vi "Main On Load Action VI.vi"(8 "error in (no error)":errorcluster, 11 "Device Item Ref in":T1 format="%.0x") -> (0 "error out":errorcluster, 3 "Device Item Ref out":T1 format="%.0x")   [LabVIEW 2011, in "Engine Sim System Explorer.lvlib"]
uses:
  Engine Sim System Explorer.lvlib
  <vilib>/NI Veristand/Custom Device API/Custom Device API.lvlib
  <vilib>/NI Veristand/Custom Device API/Custom Device Loop Type.ctl
  <vilib>/NI Veristand/Custom Device API/Custom Device Channel Type.ctl
  <vilib>/NI Veristand/Custom Device API/Custom Device Channel.ctl
  Shared/Engine Simulation Global.vi
  Engine Simulation Shared.lvlib
  <vilib>/NI Veristand/Custom Device API/Get Item Property (Dependent File).vi
  <vilib>/NI Veristand/Custom Device API/Set Item Property (Path).vi
  <vilib>/NI Veristand/Custom Device Tools/Custom Device Utility Library/Custom Device Utility Library.lvlib
  <vilib>/NI Veristand/Custom Device Tools/Custom Device Utility Library/NI VeriStand - Search for Item by GUID.vi
  <vilib>/NI Veristand/Custom Device API/Get Item Property (Boolean).vi
  <vilib>/NI Veristand/Custom Device API/Get Item Property (Dependent Node Pointer).vi
  <vilib>/NI Veristand/Custom Device API/Custom Device Execution Mode.ctl
  <vilib>/NI Veristand/Custom Device API/Path Type.ctl
  <vilib>/NI Veristand/Custom Device API/Path Specification.ctl
  <vilib>/NI Veristand/Custom Device API/Custom Device Supported Target.ctl
  <vilib>/NI Veristand/Custom Device API/Custom Device Path Data.ctl
  NationalInstruments.VeriStand.SystemDefinitionAPI
  <vilib>/NI Veristand/Custom Device API/Custom Device Item Ref.ctl
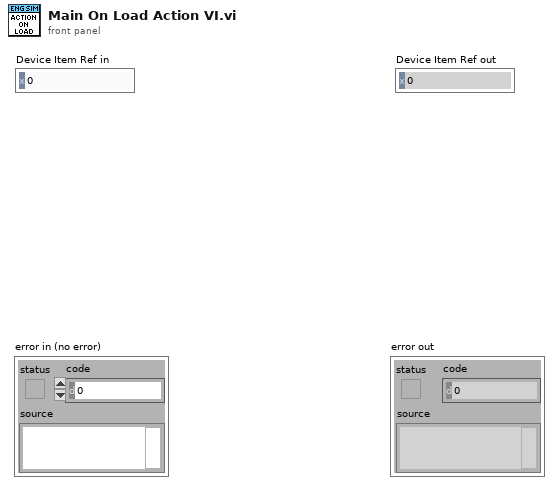
[diagram p1: front panel]
types:
  T1 = typedef "Custom Device API.lvlib/Custom Device Item Ref.ctl" = u64
  T2 = typedef "Custom Device API.lvlib/Custom Device Loop Type.ctl" = enum32{"While Loop", "Timed Loop"}
  T3 = typedef "Custom Device API.lvlib/Custom Device Channel.ctl" = cluster{"Type":T4, "Units":string, "Default Value":dbl, "Faultable":bool, "Scalable":bool}
  T4 = typedef "Custom Device API.lvlib/Custom Device Channel Type.ctl" = enum16{"Input", "Output"}
  T5 = typedef "Custom Device API.lvlib/Path Type.ctl" = enum16{"Absolute", "To Base", "To Common Data Dir", "To Application Data Dir"}
  T6 = typedef "Custom Device API.lvlib/Custom Device Supported Target.ctl" = enum16{"All", "PharLap", "VxWorks", "Windows", "PharLap & Windows", "PharLap & VxWorks", "VxWorks & Windows"}
  T7 = typedef "Custom Device API.lvlib/Custom Device Execution Mode.ctl" = enum16{"Asynchronous", "Inline HW Interface", "Inline Model Interface", "Inline Timing and Sync", "Asynchronous Timing and Sync"}
  T8 = typedef "Custom Device API.lvlib/Dependent File Optional Info.ctl" = cluster{"Version":string, "RTDestination":path, "ForceDownload":bool, "SupportedTarget":string, "MD5":string}
  T9 = typedef "Custom Device API.lvlib/Custom Device Path Data.ctl" = cluster{"SupportedTarget":T6, "Source":T10, "RT Destination":path}
  T10 = typedef "Custom Device API.lvlib/Path Specification.ctl" = cluster{"Path":path, "Type":T5}
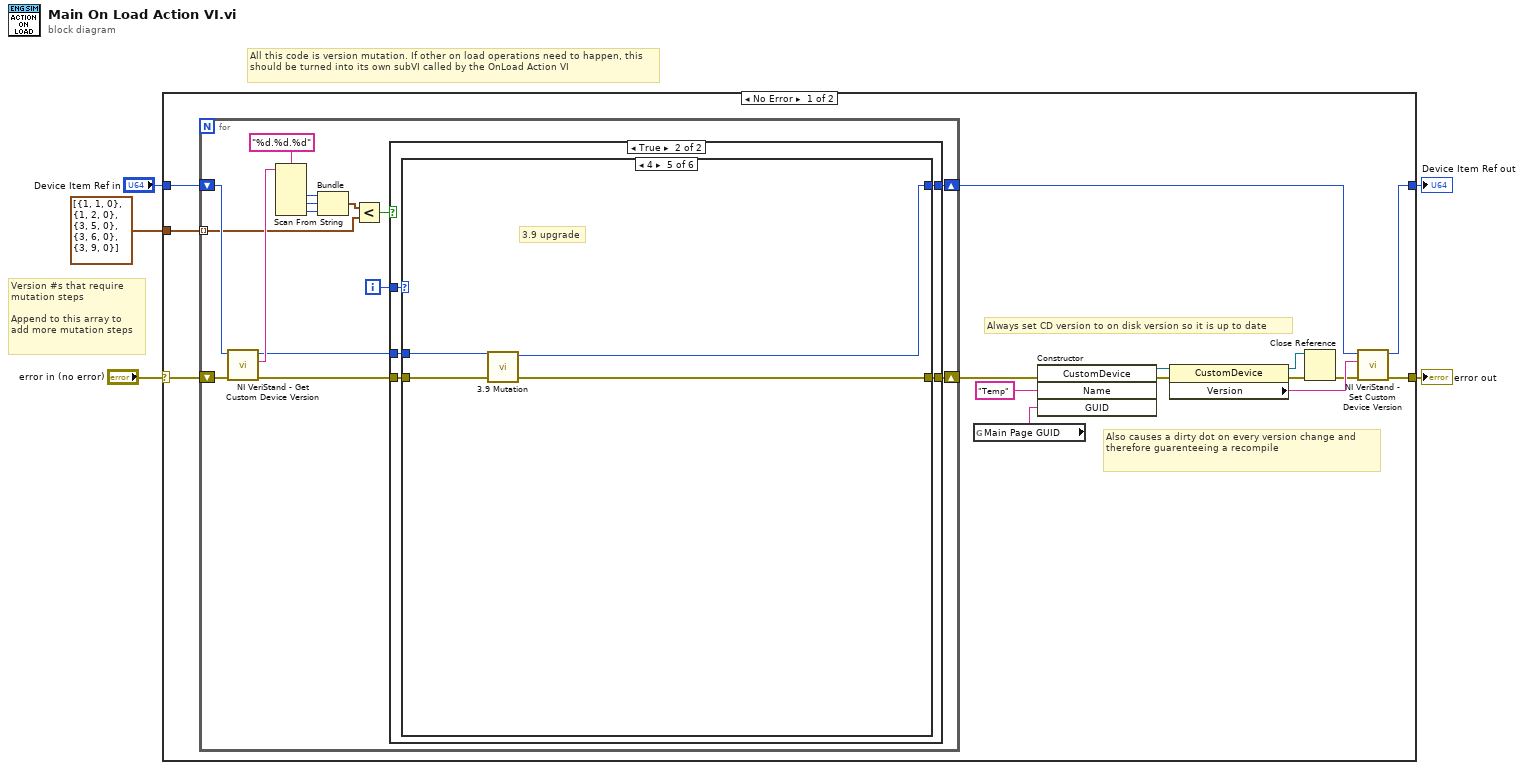
[diagram p0: block diagram]
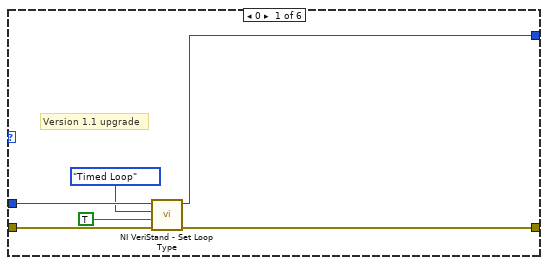
[diagram p3: hidden frame]
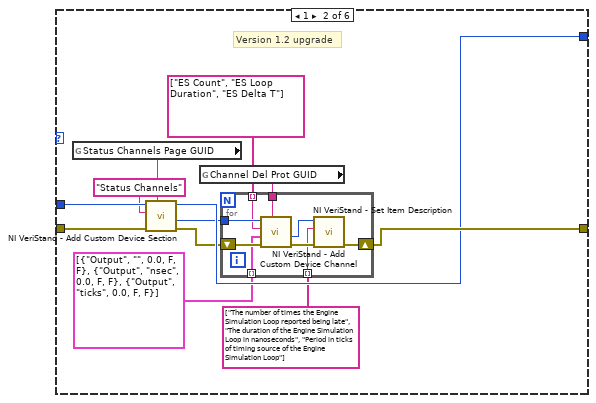
[diagram p4: hidden frame]
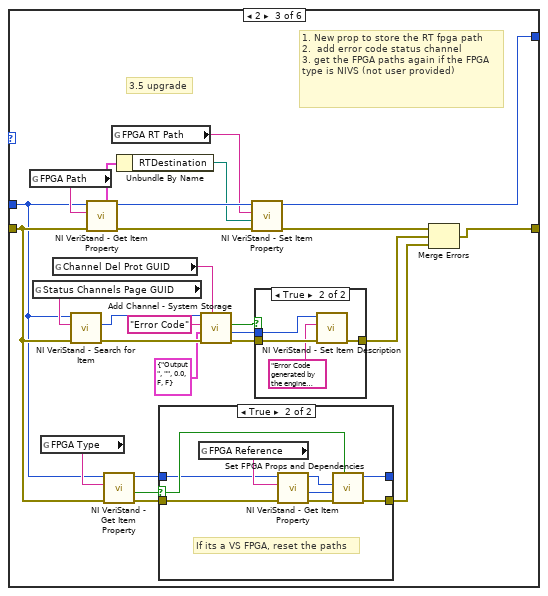
[diagram p5: hidden frame]
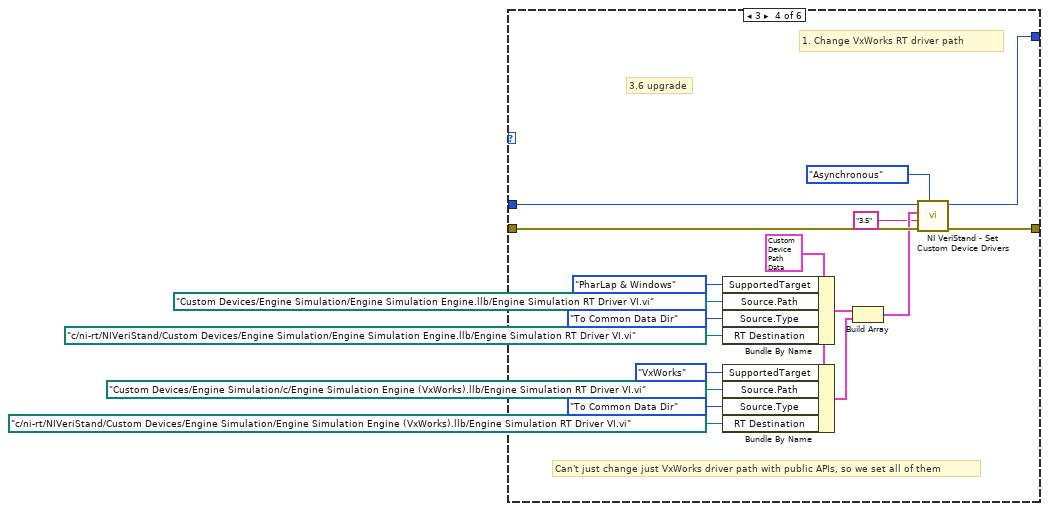
[diagram p8: hidden frame]
diagram:
  # "All this code is version mutation. If other on load operations need to happen, this should be turned into its own subVI called by the OnLoad Action VI"
  # "Version #s that require\nmutation steps\n\nAppend to this array to\nadd more mutation steps"
  n1 = case shown="No Error" "error in (no error)" {
    selector: "error in (no error)" -> [w19 w137]
    tunnel: [w9 w137] -> w4
    tunnel: "Device Item Ref in" -> [w18 w136]
    tunnel: [w7 w136] -> w2
    tunnel: cluster{i32, i32, i32}[] [{1, 1, 0}, {1, 2, 0}, {3, 5, 0}, {3, 6, 0}, {3, 9, 0}] -> [w20 _]
    frame No Error {
      # "Also causes a dirty dot on every version change and therefore guarenteeing a recompile"
      # "Always set CD version to on disk version so it is up to date"
      n2 = for {
        tunnel: w20 -> [w22] mode=indexing
        shift-right: [w26] -> w10
        shift-left: w19 -> [w31]
        shift-right: [w24] -> w8
        shift-left: w18 -> [w30]
        i -> [w23]
        n3 = call <vilib>:"NI VeriStand - Get Custom Device Version.vi"("error in (no error)"=w31, "Device Ref in"=w30) -> ("error out"=w27:errorcluster, "Value"=w29:string, "Device Ref out"=w25:T1)  [unwired: 7 in]
        n4 = Scan From String(format string="%d.%d.%d", input string=w29) -> (output 1=w33:i32, output 2=w34:i32, output 3=w21:i32)  [unwired: 5 in, 3 out]
        n5 = Bundle(w33, w34, w21) -> (w35:cluster{i32, i32, i32})  [unwired: 1 in]
        n6 = Less?(x=w35, y=w22) -> (x < y?=w28:bool)
        n7 = case shown="True" w28 {
          tunnel: w27 -> [w37 w42]
          tunnel: [w37 w41] -> w26
          tunnel: w25 -> [w36 w38]
          tunnel: [w36 w39] -> w24
          tunnel: w23 -> [_ w40]
          frame False {
          }
          frame True {
            n8 = case shown="4" w40 {
              tunnel: w42 -> [w48 w59 w76 w126 w133 w135]
              tunnel: [w45 w60 w70 w129 w131 w135] -> w41
              tunnel: [w46 w56 w89 w128 w130 w134] -> w39
              tunnel: w38 -> [w47 w58 w72 w127 w132 w134]
              frame 0 {
                # "Version 1.1 upgrade"
                n9 = call <vilib>:"NI VeriStand - Set Loop Type.vi"("error in (no error)"=w48, "Use Device Clock (Timed Loops only)"=TRUE, "Loop type"=Custom_Device_Loop_Type."Timed Loop", "Device Ref in"=w47) -> ("error out"=w45:errorcluster, "Device Ref out"=w46:T1)  [unwired: 6 in]
              }
              frame 1 {
                # "Version 1.2 upgrade"
                n10 = global read "Engine Simulation Global.vi" "Status Channels Page GUID"() -> (w49:string)
                n11 = call <vilib>:"NI VeriStand - Add Custom Device Section.vi"("GUID (Default Section)"=w49, "error in (no error)"=w59, "Section Name"="Status Channels", "Parent Ref in"=w58) -> ("error out"=w54:errorcluster, "Section Ptr"=w55:T1, "Parent Ref out"=w56:T1)  [unwired: 4 in, 1 out]
                n12 = global read "Engine Simulation Global.vi" "Channel Del Prot GUID"() -> (w52:string)
                n13 = for {
                  tunnel: w55 -> [w69]
                  shift-right: [w63] -> w60
                  shift-left: w54 -> [w68]
                  tunnel: T3[] [{"Type"=enum."Output", "Units"="", "Default Value"=0.0, "Faultable"=FALSE, "Scalable"=FALSE}, {"Type"=enum."Output", "Units"="nsec", "Default Value"=0.0, "Faultable"=FALSE, "Scalable"=FALSE}, {"Type"=enum."Output", "Units"="ticks", "Default Value"=0.0, "Faultable"=FALSE, "Scalable"=FALSE}] -> [w67] mode=indexing
                  tunnel: w52 -> [w66]
                  tunnel: string[] ["ES Count", "ES Loop Duration", "ES Delta T"] -> [w65] mode=indexing
                  tunnel: string[] ["The number of times the Engine Simulation Loop reported being late", "The duration of the Engine Simulation Loop in nanoseconds", "Period in ticks of timing source of the Engine Simulation Loop"] -> [w62] mode=indexing
                  n14 = call <vilib>:"NI VeriStand - Add Custom Device Channel.vi"("GUID (Default Channel)"=w66, "error in (no error)"=w68, "Channel"=w67, "Channel Name"=w65, "Parent Ref in"=w69) -> ("error out"=w64:errorcluster, "Channel Ref"=w61:T1)  [unwired: 3 in, 2 out]
                  n15 = call <vilib>:"NI VeriStand - Set Item Description.vi"("error in (no error)"=w64, "Description"=w62, "Item Ref in"=w61) -> ("error out"=w63:errorcluster)  [unwired: 6 in, 2 out]
                }
              }
              frame 2 {
                # "1. New prop to store the RT fpga path\n2.  add error code status channel\n3. get the FPGA paths again if the FPGA type is NIVS (not user provided)"
                # "3.5 upgrade"
                n16 = global read "Engine Simulation Global.vi" "FPGA Path"() -> (w95:string)
                n17 = global read "Engine Simulation Global.vi" "Status Channels Page GUID"() -> (w88:string)
                n18 = global read "Engine Simulation Global.vi" "FPGA Type"() -> (w80:string)
                n19 = global read "Engine Simulation Global.vi" "Channel Del Prot GUID"() -> (w84:string)
                n20 = call-poly <vilib>:"NI VeriStand - Search for Item.vi"("error in"=w76, "Item GUID"=w88, "Section Ref in"=w72) -> ("error out"=w87:errorcluster, "Item Ref"=w81:T1)  [unwired: 5 in, 2 out]
                n21 = call-poly <vilib>:"NI VeriStand - Get Item Property.vi"("error in (no error)"=w76, "Property Name"=w95, "Item Ref in"=w72) -> ("error out"=w93:errorcluster, "Item Ref out"=w92:T1, "OptionalInfo"=w94:T8)  [unwired: 4 in, 2 out]
                n22 = call-poly <vilib>:"NI VeriStand - Get Item Property.vi"("error in (no error)"=w76, "Property Name"=w80, "Item Ref in"=w72) -> ("error out"=w78:errorcluster, "Value"=w79:bool, "Item Ref out"=w77:T1)  [unwired: 5 in, 1 out]
                n23 = global read "Engine Simulation Global.vi" "FPGA RT Path"() -> (w91:string)
                n24 = Unbundle By Name(w94) -> ("RTDestination"=w90:path)
                n25 = case shown="True" w79 {
                  selector: w79 -> [_ w109]
                  tunnel: w78 -> [w102 w106]
                  tunnel: w77 -> [w101 w105]
                  tunnel: [w102 w104] -> w73
                  tunnel: [w101 w103] -> _
                  frame False {
                  }
                  frame True {
                    # "If its a VS FPGA, reset the paths"
                    n26 = global read "Engine Simulation Global.vi" "FPGA Reference"() -> (w111:string)
                    n27 = call-poly <vilib>:"NI VeriStand - Get Item Property.vi"("error in (no error)"=w106, "Property Name"=w111, "Item Ref in"=w105) -> ("error out"=w110:errorcluster, "Dependent Node Ref"=w107:T1, "Item Ref out"=w108:T1)  [unwired: 5 in, 1 out]
                    n28 = call "Set FPGA Props and Dependencies.vi"("VS FPGA?"=w109, "error in (no error)"=w110, "FPGA Ref"=w107, "CD Ref in"=w108) -> ("error out"=w104:errorcluster, "CD Ref out"=w103:T1)  [unwired: 6 in]
                  }
                }
                n29 = call "Add Channel - System Storage.vi"("GUID (Default Channel)"=w84, "error in (no error)"=w87, "Channel"=T3 {"Type"=enum."Output", "Units"="", "Default Value"=0.0, "Faultable"=FALSE, "Scalable"=FALSE}, "Channel Name"="Error Code", "Device Item Ref"=w81) -> ("error out"=w83:errorcluster, "Device Item Ref"=w82:T1, "Newly Created?"=w71:bool)  [unwired: 3 in, 1 out]
                n30 = call-poly <vilib>:"NI VeriStand - Set Item Property.vi"("error in (no error)"=w93, "Value"=w90, "Property Name"=w91, "Item Ref in"=w92) -> ("error out"=w75:errorcluster, "Item Ref out"=w89:T1)  [unwired: 5 in, 1 out]
                n31 = case shown="True" w71 {
                  tunnel: w83 -> [w96 w100]
                  tunnel: w82 -> [_ w99]
                  tunnel: [w96 w97] -> w74
                  frame False {
                  }
                  frame True {
                    n32 = call <vilib>:"NI VeriStand - Set Item Description.vi"("error in (no error)"=w100, "Description"="Error Code generated by the engine simulation cusom device. A non zero value could indicate failure." ("Channel Name"), "Item Ref in"=w99) -> ("error out"=w97:errorcluster)  [unwired: 6 in, 2 out]
                  }
                }
                n33 = Merge Errors(w75, w74, w73) -> (w70:errorcluster)
              }
              frame 3 {
                w116 = T9 {"SupportedTarget"=enum."All", "Source"={"Path"=path "", "Type"=enum."Absolute"}, "RT Destination"=path ""} ("Driver VI Path")
                # "Can't just change just VxWorks driver path with public APIs, so we set all of them"
                # "1. Change VxWorks RT driver path"
                # "3.6 upgrade"
                n34 = Bundle By Name(cluster=w116, "SupportedTarget"=Custom_Device_Supported_Target."PharLap & Windows", "Source.Path"=path "Custom Devices/Engine Simulation/Engine Simulation Engine.llb/Engine Simulation RT Driver VI.vi", "Source.Type"=Path_Type."To Common Data Dir", "RT Destination"=path "c:/ni-rt/NIVeriStand/Custom Devices/Engine Simulation/Engine Simulation Engine.llb/Engine Simulation RT Driver VI.vi") -> (w115:T9)
                n35 = Bundle By Name(cluster=w116, "SupportedTarget"=Custom_Device_Supported_Target."VxWorks", "Source.Path"=path "Custom Devices/Engine Simulation/c/Engine Simulation Engine (VxWorks).llb/Engine Simulation RT Driver VI.vi", "Source.Type"=Path_Type."To Common Data Dir", "RT Destination"=path "c:/ni-rt/NIVeriStand/Custom Devices/Engine Simulation/Engine Simulation Engine (VxWorks).llb/Engine Simulation RT Driver VI.vi") -> (w114:T9)
                n36 = Build Array(w115, w114) -> (w113:T9[])
                n37 = call <vilib>:"NI VeriStand - Set Custom Device Drivers.vi"("Execution mode"=Custom_Device_Execution_Mode."Asynchronous", "error in (no error)"=w126, "Version"="3.5", "Driver VI"=w113, "Device Ref in"=w127) -> ("error out"=w129:errorcluster, "Device Ref out"=w128:T1)  [unwired: 5 in]
              }
              frame 4 {
                # "3.9 upgrade"
                n38 = call "3.9 Mutation.vi"("error in (no error)"=w133, "Device Ref out"=w132) -> ("error out"=w131:errorcluster, "Device Ref out"=w130:T1)  [unwired: 8 in]
              }
              frame Default {
              }
            }
          }
        }
      }
      n39 = global read "Engine Simulation Global.vi" "Main Page GUID"() -> (w6:string)
      n40 = constructor class="CustomDevice"(error in=w10, "Name"="Temp", "GUID"=w6) -> (reference out=w16:refnum<k24>, error out=w15:errorcluster)  [unwired: 2 in, 3 out]
      n41 = property class="CustomDevice"(reference=w16, error in=w15) -> (reference out=w13:refnum<k24>, error out=w14:errorcluster, "Version"=w12:string)
      n42 = Close Reference(reference=w13, error in (no error)=w14) -> (error out=w11:errorcluster)
      n43 = call <vilib>:"NI VeriStand - Set Custom Device Version.vi"("error in (no error)"=w11, "Value"=w12, "Device Ref in"=w8) -> ("error out"=w9:errorcluster, "Device Ref out"=w7:T1)  [unwired: 7 in]
    }
    frame Error {
    }
  }
  "error out" <- w4
  "Device Item Ref out" <- w2
